vi "ReadConfigFile.vi"() -> (3 "Config":T1 {"Max reports to save" min=1})   [LabVIEW 2020, in "DependencyViewer.lvlib"]
uses:
  DependencyViewer/DependencyViewer.lvlib
  Settings.ctl
  DependencyConfiguration.ctl
  FilterOptions.ctl
  <vilib>/Utility/sysdir.llb/System Directory Type.ctl
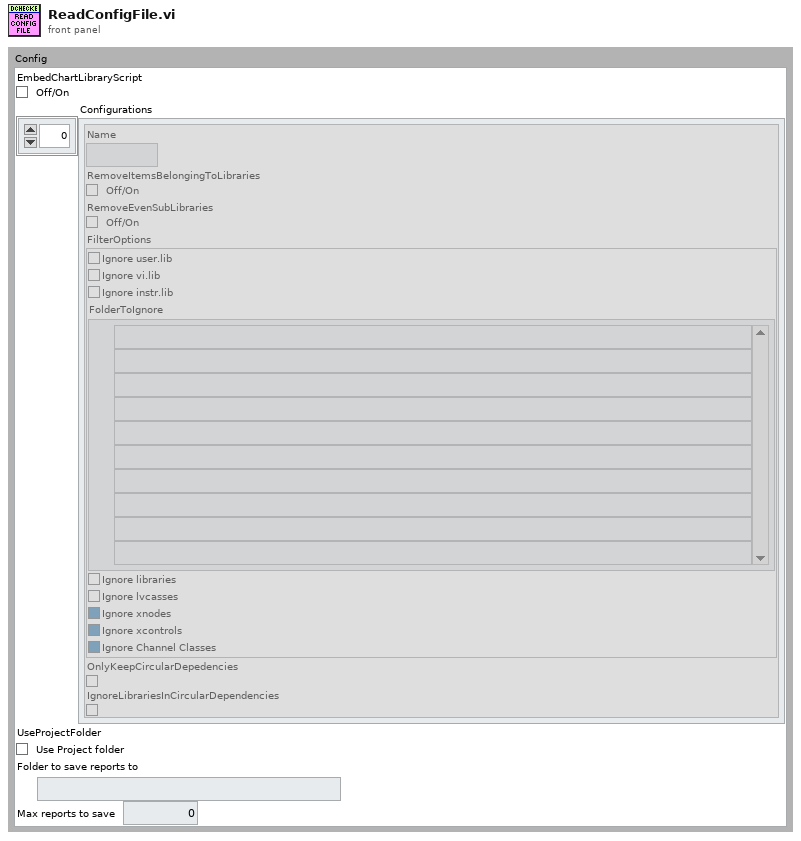
[diagram p1: front panel]
types:
  T1 = typedef "DependencyViewer.lvlib/Settings.ctl" = cluster{"EmbedChartLibraryScript":bool, "Configurations":T2[], "UseProjectFolder":bool, "Folder to save reports to":path, "Max reports to save":u8}
  T2 = typedef "DependencyViewer.lvlib/DependencyConfiguration.ctl" = cluster{"Name":string, "RemoveItemsBelongingToLibraries":bool, "RemoveEvenSubLibraries":bool, "FilterOptions":T3, "OnlyKeepCircularDepedencies":bool, "IgnoreLibrariesInCircularDependencies":bool}
  T3 = typedef "DependencyViewer.lvlib/FilterOptions.ctl" = cluster{"Ignore user.lib":bool, "Ignore vi.lib":bool, "Ignore instr.lib":bool, "FolderToIgnore":path[], "Ignore libraries":bool, "Ignore lvcasses":bool, "Ignore xnodes":bool, "Ignore xcontrols":bool, "Ignore Channel Classes":bool}
  T4 = typedef "System Directory Type.ctl" = i32
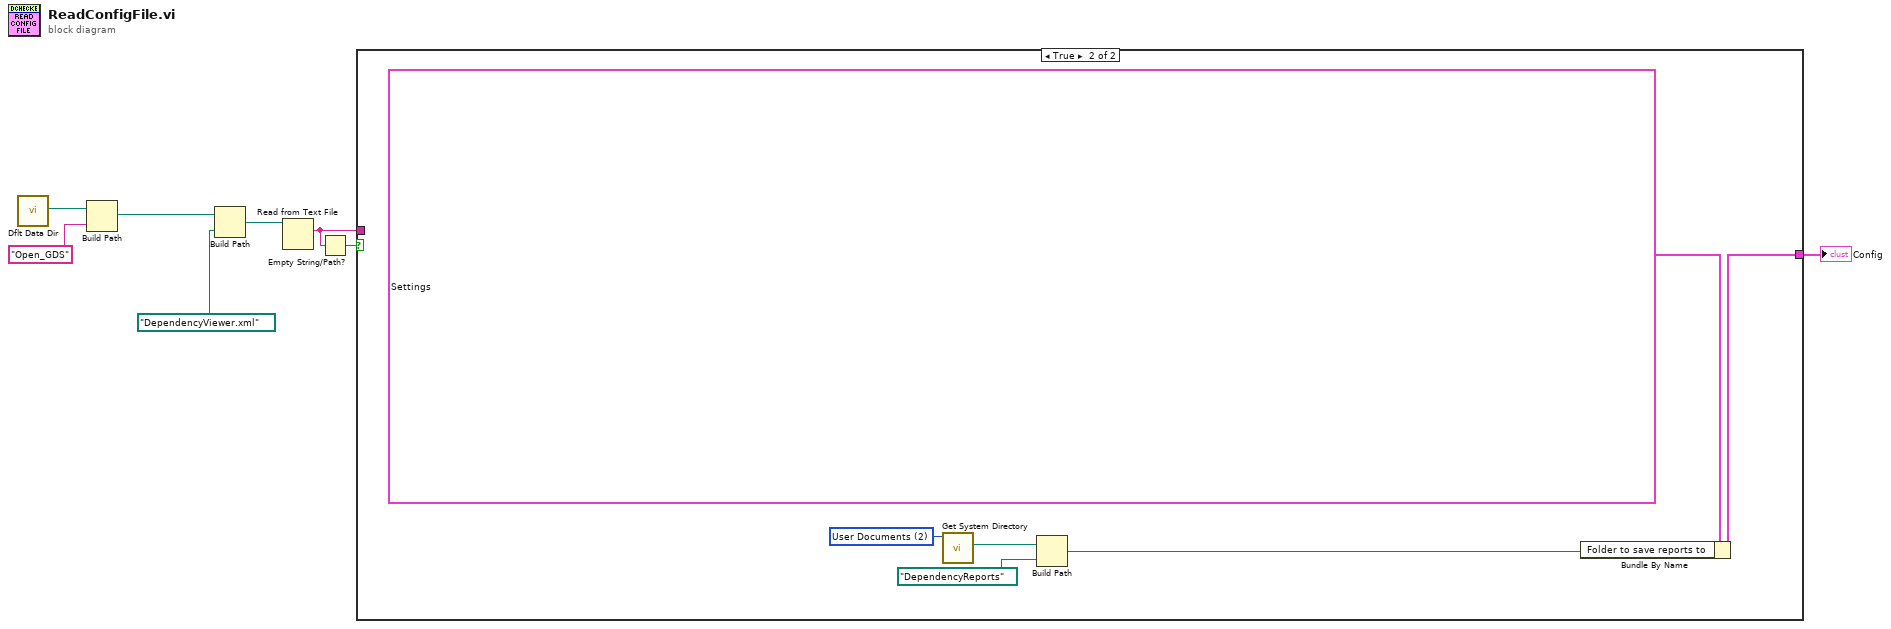
[diagram p0: block diagram]
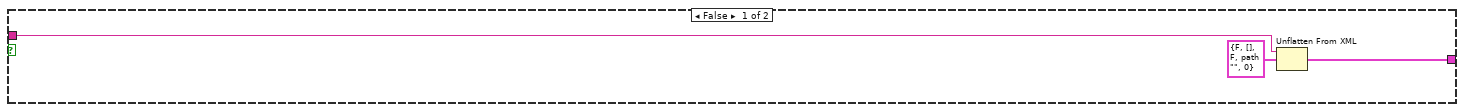
[diagram p2: hidden frame]
diagram:
  n1 = call <vilib>:"Dflt Data Dir.vi"() -> ("App:Default Data Directory"=w5:path)
  n2 = Build Path(base path=w5, name or relative path="Open_GDS") -> (appended path=w1:path)
  n3 = Build Path(base path=w1, name or relative path=path "DependencyViewer.xml") -> (appended path=w2:path)
  n4 = Read from Text File(file (use dialog)=w2) -> (text=w7:string)  [unwired: 3 in, 3 out]
  n5 = Empty String/Path?(string/path=w7) -> (empty?=w6:bool)
  n6 = case shown="True" w6 {
    tunnel: [w10 w16] -> w8
    tunnel: w7 -> [w9 _]
    frame False {
      n7 = Unflatten From XML(xml string=w9, type=T1 {"EmbedChartLibraryScript"=FALSE, "Configurations"=[], "UseProjectFolder"=FALSE, "Folder to save reports to"=path "", "Max reports to save"=0}) -> (value=w10:T1)  [unwired: 1 in, 1 out]
    }
    frame True {
      w15 = T4 2 items=["User Home"=0, "User Desktop"=1, "User Documents"=2, "User Application Data"=3, "User Preferences"=4, "User Temporary"=5, "Public Documents"=6, "Public Application Data"=7, "Public Preferences"=8, "Public Cache"=13, "System Core Libraries"=9, "System Installed Libraries"=10, "Application Files"=11, "Boot Volume Root"=12] ("system directory type")
      n8 = call <vilib>:"Get System Directory.vi"("system directory type"=w15) -> ("system directory"=w14:path)  [unwired: 10 in]
      n9 = Build Path(base path=w14, name or relative path=path "DependencyReports") -> (appended path=w12:path)
      n10 = Bundle By Name(cluster=T1 {"EmbedChartLibraryScript"=FALSE, "Configurations"=[{"Name"="All classes", "RemoveItemsBelongingToLibraries"=FALSE, "RemoveEvenSubLibraries"=FALSE, "FilterOptions"={"Ignore user.lib"=FALSE, "Ignore vi.lib"=FALSE, "Ignore instr.lib"=FALSE, "FolderToIgnore"=[], "Ignore libraries"=TRUE, "Ignore lvcasses"=FALSE, "Ignore xnodes"=TRUE, "Ignore xcontrols"=TRUE, "Ignore Channel Classes"=TRUE}, "OnlyKeepCircularDepedencies"=FALSE, "IgnoreLibrariesInCircularDependencies"=FALSE}, {"Name"="All libraries", "RemoveItemsBelongingToLibraries"=FALSE, "RemoveEvenSubLibraries"=FALSE, "FilterOptions"={"Ignore user.lib"=FALSE, "Ignore vi.lib"=FALSE, "Ignore instr.lib"=FALSE, "FolderToIgnore"=[], "Ignore libraries"=FALSE, "Ignore lvcasses"=TRUE, "Ignore xnodes"=TRUE, "Ignore xcontrols"=TRUE, "Ignore Channel Classes"=TRUE}, "OnlyKeepCircularDepedencies"=FALSE, "IgnoreLibrariesInCircularDependencies"=FALSE}, {"Name"="All classes with circular dependencies", "RemoveItemsBelongingToLibraries"=FALSE, "RemoveEvenSubLibraries"=FALSE, "FilterOptions"={"Ignore user.lib"=FALSE, "Ignore vi.lib"=FALSE, "Ignore instr.lib"=FALSE, "FolderToIgnore"=[], "Ignore libraries"=TRUE, "Ignore lvcasses"=FALSE, "Ignore xnodes"=TRUE, "Ignore xcontrols"=TRUE, "Ignore Channel Classes"=TRUE}, "OnlyKeepCircularDepedencies"=TRUE, "IgnoreLibrariesInCircularDependencies"=FALSE}, {"Name"="All libraries with circular dependencies", "RemoveItemsBelongingToLibraries"=FALSE, "RemoveEvenSubLibraries"=FALSE, "FilterOptions"={"Ignore user.lib"=FALSE, "Ignore vi.lib"=FALSE, "Ignore instr.lib"=FALSE, "FolderToIgnore"=[], "Ignore libraries"=FALSE, "Ignore lvcasses"=TRUE, "Ignore xnodes"=TRUE, "Ignore xcontrols"=TRUE, "Ignore Channel Classes"=TRUE}, "OnlyKeepCircularDepedencies"=TRUE, "IgnoreLibrariesInCircularDependencies"=FALSE}], "UseProjectFolder"=FALSE, "Folder to save reports to"=path "", "Max reports to save"=20}, "Folder to save reports to"=w12) -> (w16:T1)
    }
  }
  "Config" <- w8
